vi "Drivetrain Past Target.vi"(9 "Target Y":dbl, 10 "Target X":dbl, 11 "Reset":bool) -> (3 "Past Target?":bool)   [LabVIEW 2014]
uses:
  Robot Global Data.vi
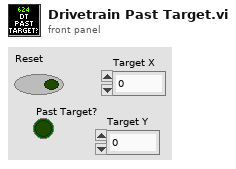
[diagram p1: front panel]
types:
  T1 = typedef "Encoder Values.ctl" = cluster{"Distance":dbl, "Speed":dbl, "Ticks":dbl}
  T2 = cluster{"Left Encoder":T1, "Center Encoder":T1, "Right Encoder":T1}
  T3 = typedef "Drivetrain Control.ctl" = cluster{"Mode":T4, "Steer":dbl, "Y":dbl, "Heading Target":dbl, "Strafe X":dbl, "Y Target":dbl, "Strafe Target":dbl}
  T4 = typedef "Drivetrain Mode.ctl" = enum16{"Manual", "Gyro Steer", "Vision Steer", "Drive Distance"}
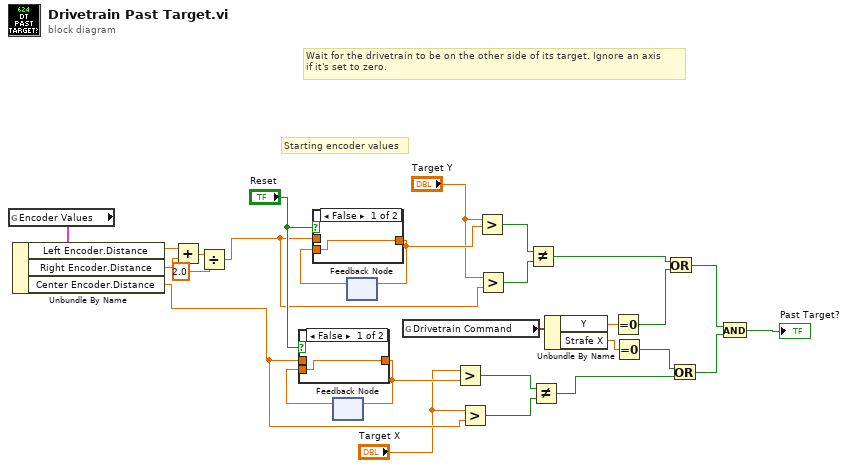
[diagram p0: block diagram]
diagram:
  # "Wait for the drivetrain to be on the other side of its target. Ignore an axis\nif it's set to zero."
  # "Starting encoder values"
  n1 = global read "Robot Global Data.vi" "Encoder Values"() -> (w28:T2)
  n2 = Unbundle By Name(w28) -> ("Left Encoder.Distance"=w24:dbl, "Right Encoder.Distance"=w23:dbl, "Center Encoder.Distance"=w16:dbl)
  n3 = Add(x=w24, y=w23) -> (x+y=w22:dbl)
  n4 = Divide(x=w22, y=2.0) -> (x/y=w14:dbl)
  n5 = feedback #1() -> (w20:dbl)  [unwired: 1 in]
  n6 = case shown="False" "Reset" {
    tunnel: w16 -> [_ w30]
    tunnel: [w29 w30] -> w17
    tunnel: w20 -> [w29 _]
    frame False {
    }
    frame True {
    }
  }
  n7 = feedback-in #1(w17) -> ()
  n8 = feedback #2() -> (w19:dbl)  [unwired: 1 in]
  n9 = case shown="False" "Reset" {
    tunnel: [w31 w32] -> w15
    tunnel: w19 -> [w31 _]
    tunnel: w14 -> [_ w32]
    frame False {
    }
    frame True {
    }
  }
  n10 = feedback-in #2(w15) -> ()
  n11 = global read "Robot Global Data.vi" "Drivetrain Command"() -> (w27:T3)
  n12 = Greater?(x="Target X", y=w17) -> (0:w11:bool)
  n13 = Greater?(x="Target X", y=w16) -> (0:w10:bool)
  n14 = Greater?(x="Target Y", y=w15) -> (0:w13:bool)
  n15 = Greater?(x="Target Y", y=w14) -> (0:w12:bool)
  n16 = Not Equal?(x=w13, y=w12) -> (x != y?=w8:bool)
  n17 = Not Equal?(x=w11, y=w10) -> (x != y?=w9:bool)
  n18 = Unbundle By Name(w27) -> ("Y"=w25:dbl, "Strafe X"=w26:dbl)
  n19 = Equal To 0?(x=w25) -> (x = 0?=w6:bool)
  n20 = Equal To 0?(x=w26) -> (x = 0?=w7:bool)
  n21 = Or(x=w8, y=w6) -> (x .or. y?=w5:bool)
  n22 = Or(x=w7, y=w9) -> (x .or. y?=w4:bool)
  n23 = And(x=w5, y=w4) -> (x .and. y?=→"Past Target?":bool)
